vi "Insert Subroutine.vi"(0 "Custom Type Test Executive in":refnum<class "Custom Type Test Executive.lvclass">, 1 "Parent ID":string, 5 "Name":string, 9 "File Path":string, 11 "error in (no error)":errorcluster, 12 "Insertion Index":i32=-1, 13 "Path Builder":refnum<class "IPath Builder.lvclass">, 14 "Persistence":refnum<class "IPersist.lvclass">) -> (3 "Unique ID out":string, 4 "Custom Type Test Executive out":refnum<class "Custom Type Test Executive.lvclass">, 8 "Replaced?":bool, 15 "error out":errorcluster)   [LabVIEW 2017, in "Custom Type Test Executive.lvlib" / "Custom Type Test Executive.lvclass"]
uses:
  <vilib>/gpm_packages/@cs/test-executive/Source/Custom Type Test Executive/Custom Type Test Executive/Custom Type Test Executive.lvclass
  C:/Program Files/National Instruments/LabVIEW 2017/vi.lib/gpm_packages/@cs/test-executive/Source/Test Executive/TestExecutive/Test Executive.lvclass
  <vilib>/gpm_packages/@cs/persistence/source/IPersist/IPersist.lvclass
  <vilib>/gpm_packages/@cs/test-executive/Source/Path Builder/IPath Builder/IPath Builder.lvclass
  <vilib>/gpm_packages/@cs/test-executive/Source/Test Executive/ITestExecutive/ITest Executive.lvclass
  <vilib>/gpm_packages/@cs/test-executive/Source/Custom Type Test Executive/Subroutine/Subroutine.lvclass
  <vilib>/gpm_packages/@cs/data-type-serializer/source/Boolean/Boolean.lvclass/Boolean.ctl
  <vilib>/gpm_packages/@cs/data-type-serializer/source/String/String.lvclass/String.ctl
  <vilib>/gpm_packages/@cs/test-executive/Source/Custom Type Test Executive/Test Executive Data Type/Test Executive.lvclass/Test Executive.ctl
  <vilib>/gpm_packages/@cs/test-executive/Source/Test Executive/TestExecutive/Test Executive.lvclass/Test Executive.ctl
  <vilib>/gpm_packages/@cs/test-executive/Source/Custom Type Test Executive/Persistence Data Type/Persistence.lvclass/Persistence.ctl
  <vilib>/gpm_packages/@cs/test-executive/Source/Custom Type Test Executive/Path Builder Data Type/Path Builder.lvclass/Path Builder.ctl
  bf01cd08-8183-47d8-84d8-b3c1fc62e279.vi
  fa034ab8-2756-433a-8a58-ebe5b51d12f0.vi
  bf8ca4d2-c0bb-42dd-8b81-6217ed55653d.vi
  5ccc8c70-6791-4b3c-8d27-b93e5551dbd8.vi
  9fe0d12a-4a70-45e6-bcc1-56eebd74c584.vi
  9126d2dd-f8a7-409e-bc78-72e360319254.vi
  00cde055-f706-4b27-a7ba-fedab2966742.vi
  4d8faee1-13ea-4f80-b0b7-62e2134826e5.vi
  <vilib>/gpm_packages/@cs/test-executive/Source/Custom Type Test Executive/Persistence Data Type/Persistence.lvclass
  <vilib>/gpm_packages/@cs/data-type-serializer/source/String/String.lvclass
  <vilib>/gpm_packages/@cs/test-executive/Source/Custom Type Test Executive/Path Builder Data Type/Path Builder.lvclass
  <vilib>/gpm_packages/@cs/data-type-serializer/source/Boolean/Boolean.lvclass
  <vilib>/gpm_packages/@cs/test-executive/Source/Custom Type Test Executive/Test Executive Data Type/Test Executive.lvclass
  <vilib>/gpm_packages/@cs/linked-list/Source/Linked List/ILinkedList/ILinked List.lvclass
  <vilib>/gpm_packages/@cs/linked-list/Source/Linked List/Linked List Ref/Linked List Ref.lvclass
  <vilib>/gpm_packages/@cs/test-executive/Source/Test Executive/TestExecutive/Test Executive.lvclass
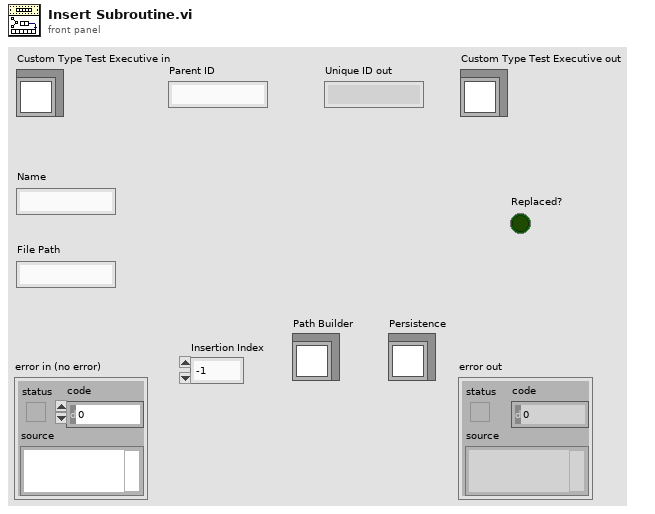
[diagram p1: front panel]
types:
  T1 = enum16{"open", "replace", "create", "open or create", "replace or create", "replace or create with confirmation"}
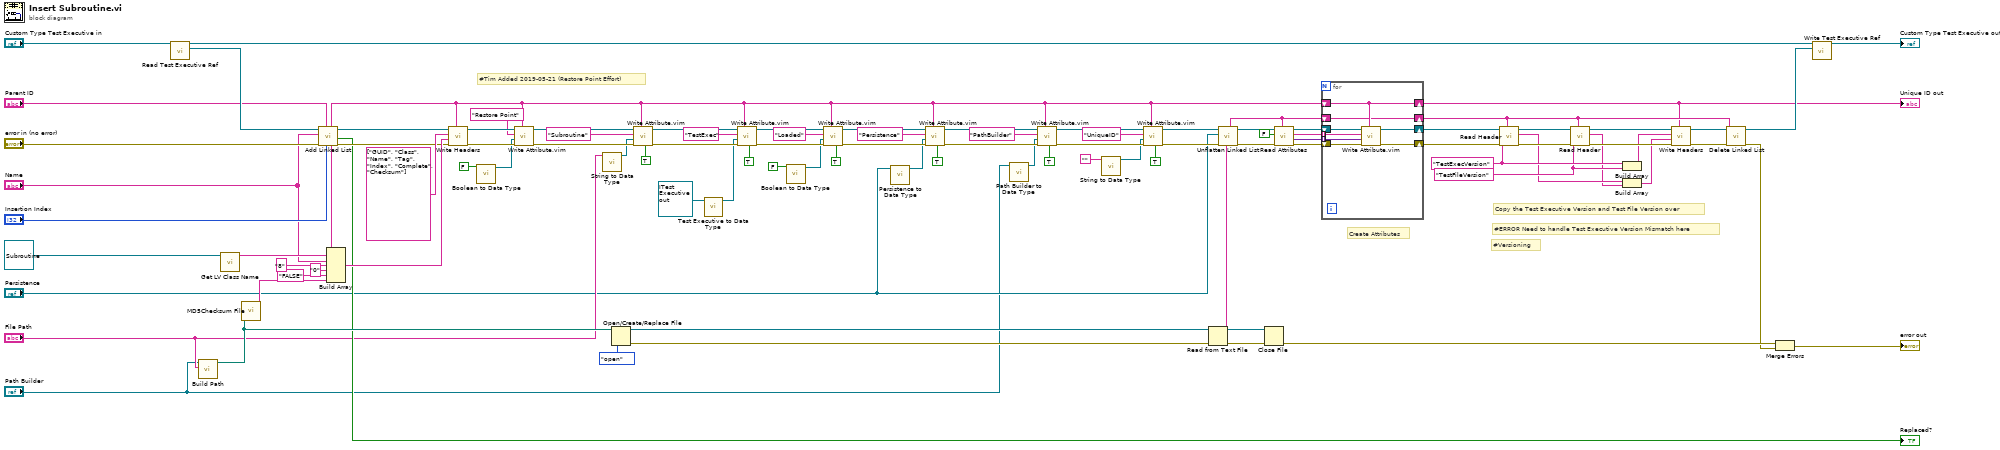
[diagram p0: block diagram]
diagram:
  w33 = "TestFileVersion" ("Header Name")
  w34 = "TestExecVersion" ("Header Name")
  # "#Versioning"
  # "#ERROR Need to handle Test Executive Version Mismatch here"
  # "Copy the Test Executive Version and Test File Version over"
  # "Create Attributes"
  # "#Tim Added 2019-05-21 (Restore Point Effort)"
  n1 = call <vilib>:"Read Test Executive Ref.vi"("Test Executive in"="Custom Type Test Executive in") -> ("Test Executive Ref"=w26:refnum<data-value>, "Test Executive out"=w25:refnum<class "Custom Type Test Executive.lvclass">)  [unwired: 9 in]
  n2 = call-dynamic "Build Path.vi"("Path"="File Path", "IPath Builder in"="Path Builder") -> ("Path"=w51:path)  [unwired: 8 in, 1 out]
  n3 = call <vilib>:"Get LV Class Name.vi"("object"=refnum<class "Subroutine.lvclass"> refnum ("Custom Type Test Executive.lvlib:Subroutine.lvclass")) -> ("class name"=w94:string)  [unwired: 9 in, 1 out]
  n4 = call <vilib>:"MD5Checksum File.vi"("Path"=w51) -> ("MD5 message-digest"=w81:string)  [unwired: 9 in, 1 out]
  n5 = call <vilib>:"Add Linked List.vi"("Insertion Index"="Insertion Index", "Parent ID"="Parent ID", "error in (no error)"="error in (no error)", "Name"="Name", "Linked List Ref"=w26) -> ("error out"=w95:errorcluster, "Replaced?"=→"Replaced?":bool, "Linked List Ref out"=w96:refnum<data-value>, "Linked List ID out"=w44:string)  [unwired: 3 in]
  n6 = Build Array(w44, w94, "Name", "8" ("Tag"), "0" ("element"), "FALSE" ("element"), w81) -> (w97:string[])
  n7 = call <vilib>:"Write Headers.vi"("Linked List ID"=w44, "error in (no error)"=w95, "Header Values"=w97, "Header Names"=string[] ["GUID", "Class", "Name", "Tag", "Index", "Complete", "Checksum"], "Linked List Ref"=w96) -> ("error out"=w85:errorcluster, "Linked List Ref out"=w86:refnum<data-value>)  [unwired: 5 in]
  n8 = call <vilib>:"Boolean to Data Type.vi"("Boolean"=FALSE) -> ("Boolean out"=w14:refnum<class "Boolean.lvclass">)  [unwired: 9 in, 1 out]
  n9 = call "Write Attribute.vim"("Linked List ID"=w44, "error in (no error)"=w85, "Attribute"=w14, "Attribute Name"="Restore Point", "Linked List Ref"=w86) -> ("error out"=w73:errorcluster, "Linked List Ref out"=w74:refnum<data-value>)  [unwired: 3 in, 2 out]
  n10 = call <vilib>:"String to Data Type.vi"("String"="File Path") -> ("Boolean out"=w11:refnum<class "String.lvclass">)  [unwired: 9 in, 1 out]
  n11 = Open/Create/Replace File(file path (use dialog)=w51, operation (0:open)=T1."open") -> (refnum out=w80:refnum<file>, error out=w91:errorcluster)  [unwired: 4 in, 1 out]
  n12 = call "Write Attribute.vim"("Private?"=TRUE, "Linked List ID"=w44, "error in (no error)"=w73, "Attribute"=w11, "Attribute Name"="Subroutine", "Linked List Ref"=w74) -> ("error out"=w59:errorcluster, "Linked List Ref out"=w61:refnum<data-value>)  [unwired: 2 in, 2 out]
  n13 = call <vilib>:"Test Executive to Data Type.vi"("Test Executive Ref"=refnum<data-value> refnum ("Test Executive Ref out")) -> ("Boolean out"=w9:refnum<class "Test Executive.lvclass">)  [unwired: 9 in, 1 out]
  n14 = call "Write Attribute.vim"("Private?"=TRUE, "Linked List ID"=w44, "error in (no error)"=w59, "Attribute"=w9, "Attribute Name"="TestExec", "Linked List Ref"=w61) -> ("error out"=w58:errorcluster, "Linked List Ref out"=w60:refnum<data-value>)  [unwired: 2 in, 2 out]
  n15 = call <vilib>:"Boolean to Data Type.vi"("Boolean"=FALSE) -> ("Boolean out"=w7:refnum<class "Boolean.lvclass">)  [unwired: 9 in, 1 out]
  n16 = call "Write Attribute.vim"("Private?"=TRUE, "Linked List ID"=w44, "error in (no error)"=w58, "Attribute"=w7, "Attribute Name"="Loaded", "Linked List Ref"=w60) -> ("error out"=w67:errorcluster, "Linked List Ref out"=w68:refnum<data-value>)  [unwired: 2 in, 2 out]
  n17 = call <vilib>:"Persistence to Data Type.vi"("Persistence"="Persistence") -> ("Boolean out"=w4:refnum<class "Persistence.lvclass">)  [unwired: 9 in, 1 out]
  n18 = call "Write Attribute.vim"("Private?"=TRUE ("Pointer?"), "Linked List ID"=w44, "error in (no error)"=w67, "Attribute"=w4, "Attribute Name"="Persistence", "Linked List Ref"=w68) -> ("error out"=w46:errorcluster, "Linked List Ref out"=w48:refnum<data-value>)  [unwired: 2 in, 2 out]
  n19 = call <vilib>:"Path Builder to Data Type.vi"("Path Builder"="Path Builder") -> ("Boolean out"=w1:refnum<class "Path Builder.lvclass">)  [unwired: 9 in, 1 out]
  n20 = call "Write Attribute.vim"("Private?"=TRUE ("Pointer?"), "Linked List ID"=w44, "error in (no error)"=w46, "Attribute"=w1, "Attribute Name"="PathBuilder", "Linked List Ref"=w48) -> ("error out"=w45:errorcluster, "Linked List Ref out"=w47:refnum<data-value>)  [unwired: 2 in, 2 out]
  n21 = call <vilib>:"String to Data Type.vi"("String"="") -> ("Boolean out"=w5:refnum<class "String.lvclass">)  [unwired: 9 in, 1 out]
  n22 = call "Write Attribute.vim"("Private?"=TRUE ("Pointer?"), "Linked List ID"=w44, "error in (no error)"=w45, "Attribute"=w5, "Attribute Name"="UniqueID", "Linked List Ref"=w47) -> ("error out"=w54:errorcluster, "Linked List Ref out"=w55:refnum<data-value>)  [unwired: 2 in, 2 out]
  n23 = Read from Text File(file (use dialog)=w80, error in=w91) -> (refnum out=w90:refnum<file>, text=w88:string, error out=w92:errorcluster)  [unwired: 2 in, 1 out]
  n24 = call <vilib>:"Unflatten Linked List.vi"("Flattened Linked List"=w88, "error in (no error)"=w54, "Persistence"="Persistence", "Linked List Ref"=w55) -> ("error out"=w77:errorcluster, "Linked List Ref out"=w78:refnum<data-value>, "Linked List ID out"=w52:string)  [unwired: 5 in]
  n25 = Close File(refnum=w90, error in=w92) -> (error out=w87:errorcluster)  [unwired: 1 out]
  n26 = call <vilib>:"Read Attributes.vi"("Linked List ID"=w52, "error in (no error)"=w77, "Include Private?"=FALSE, "Linked List Ref"=w78) -> ("error out"=w71:errorcluster, "Attributes"=w28:variant[], "Attribute Names out"=w70:string[], "Linked List Ref out"=w72:refnum<data-value>)  [unwired: 2 in, 2 out]
  n27 = for {
    shift-right: [w105] -> w43
    shift-left: w72 -> [w106]
    shift-right: [w103] -> w42
    shift-left: w71 -> [w104]
    shift-right: [w102] -> w15
    shift-left: w44 -> [w102]
    tunnel: w70 -> [w101] mode=indexing
    shift-right: [w100] -> w41
    shift-left: w52 -> [w100]
    tunnel: w28 -> [w99] mode=indexing
    n28 = call "Write Attribute.vim"("Linked List ID"=w102, "error in (no error)"=w104, "Attribute"=w99, "Attribute Name"=w101, "Linked List Ref"=w106) -> ("error out"=w103:errorcluster, "Linked List Ref out"=w105:refnum<data-value>)  [unwired: 3 in, 2 out]
  }
  "Unique ID out" <- w15
  n29 = call <vilib>:"Read Header.vi"("Linked List ID"=w41, "error in (no error)"=w42, "Header Name"=w34, "Linked List Ref"=w43) -> ("error out"=w39:errorcluster, "Header Value"=w31:string, "Linked List Ref out"=w40:refnum<data-value>)  [unwired: 4 in, 1 out]
  n30 = call <vilib>:"Read Header.vi"("Linked List ID"=w41, "error in (no error)"=w39, "Header Name"=w33, "Linked List Ref"=w40) -> ("error out"=w36:errorcluster, "Header Value"=w30:string, "Linked List Ref out"=w38:refnum<data-value>)  [unwired: 4 in, 1 out]
  n31 = Build Array(w34, w33) -> (w32:string[])
  n32 = Build Array(w31, w30) -> (w29:string[])
  n33 = call <vilib>:"Write Headers.vi"("Linked List ID"=w15, "error in (no error)"=w36, "Header Values"=w29, "Header Names"=w32, "Linked List Ref"=w38) -> ("error out"=w35:errorcluster, "Linked List Ref out"=w37:refnum<data-value>)  [unwired: 5 in]
  n34 = call <vilib>:"Delete Linked List.vi"("error in (no error)"=w35, "Linked List ID"=w41, "Linked List Ref"=w37) -> ("error out"=w53:errorcluster, "Linked List Ref out"=w24:refnum<data-value>)  [unwired: 7 in]
  n35 = Merge Errors(w87, w53) -> (→"error out":errorcluster)
  n36 = call <vilib>:"Write Test Executive Ref.vi"("Test Executive Ref"=w24, "Test Executive in"=w25) -> ("Test Executive out"=→"Custom Type Test Executive out":refnum<class "Custom Type Test Executive.lvclass">)  [unwired: 9 in]
